vi "Sorting_array.vi"() -> ()   [LabVIEW 2021]
panel:
  out "Output Even Number":dbl
  in  "Orignal Array":dbl[](array[numeric])
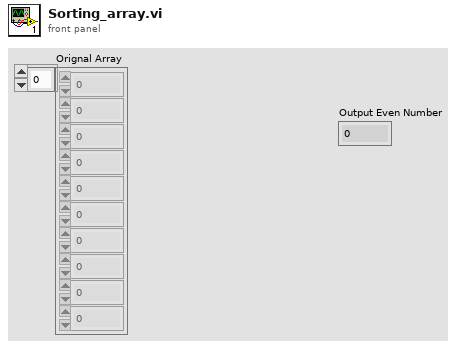
[diagram p1: front panel]
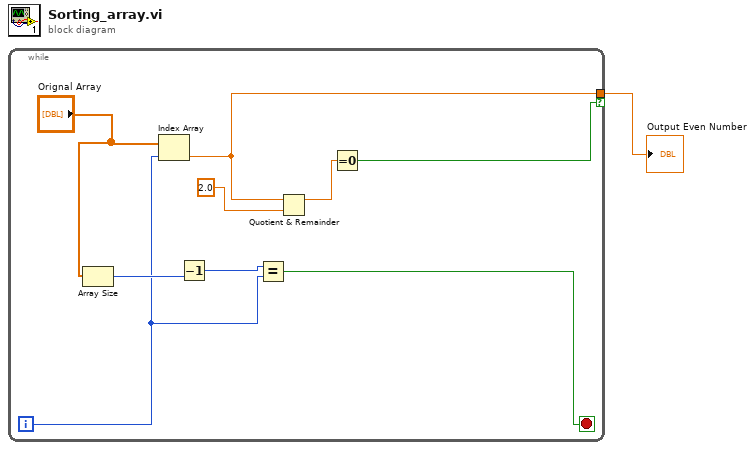
[diagram p0: block diagram]
diagram:
  n1 = while {
    tunnel: [w8] -> w1 if=w7
    i -> [w4]
    stop <- w3 stop-if-true
    n2 = Array Size(array="Orignal Array") -> (size(s)=w5:i32)
    n3 = Index Array "Index Array"(array="Orignal Array", index=w4) -> (element=w8:dbl)
    n4 = Decrement(x=w5) -> (x-1=w2:i32)
    n5 = Equal?(x=w2, y=w4) -> (x = y?=w3:bool)
    n6 = Quotient & Remainder(x=w8, y=2.0) -> (x-y*floor(x/y)=w9:dbl)  [unwired: 1 out]
    n7 = Equal To 0?(x=w9) -> (x = 0?=w7:bool)
  }
  "Output Even Number" <- w1
